vi "initialise.vi"(8 "error in (no error)":errorcluster, 11 "GenericPlugin in":refnum<class "GenericStringGenerator.lvclass">) -> (0 "error out":errorcluster, 3 "GenericPlugin out":refnum<class "GenericStringGenerator.lvclass">)   [LabVIEW 2010, in "GenericStringGenerator.lvclass"]
doc: "The dynamic dispatch-version of this VI initalises the plug-in object by allocating and initalising any dynamic resources need."
uses:
  GenericStringGenerator.lvclass
  common/classes/GenericComponent/GenericComponent/GenericComponent.lvclass
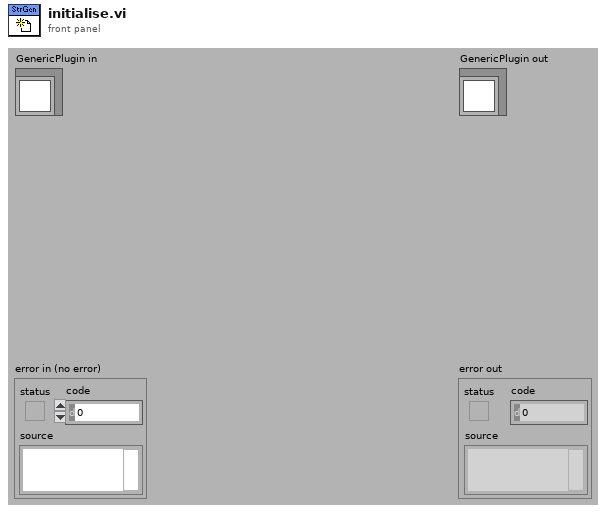
[diagram p1: front panel]
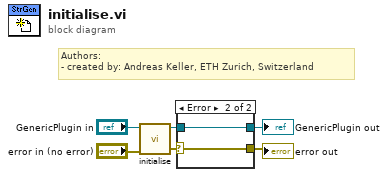
[diagram p0: block diagram]
diagram:
  # "Authors: \n- created by: Andreas Keller, ETH Zurich, Switzerland"
  n1 = call-parent "initialise.vi"("error in (no error)"="error in (no error)", "GenericPlugin in"="GenericPlugin in") -> ("error out"=w4:errorcluster, "GenericPlugin out"=w1:refnum<class "GenericStringGenerator.lvclass">)  [unwired: 8 in]
  n2 = case shown="Error" w4 {
    selector: w4 -> [w8 w10]
    tunnel: [w8 w10] -> w3
    tunnel: [w7 w9] -> w2
    tunnel: w1 -> [w7 w9]
    frame No Error {
    }
    frame Error {
    }
  }
  "error out" <- w3
  "GenericPlugin out" <- w2
